vi "transfer char run_subvi_14_2014 05 30_JWa.vi"(0 "VISA session":refnum<visa-resource-name>="GPIB0::17::INSTR", 1 "Y2 axis settings":T7={"Y2 axis on/off"=FALSE, "MINIMUM"=0.0, "MAXIMUM"=1.0, "Variable name"="Ig", "LIN or LOG axis"="LIN"} {"MAXIMUM" format="%.9f"; "MINIMUM" format="%.9f"}, 3 "LKG Path":path, 5 "Var1 sweep settings":T9={"start"=40.0, "stop"=-40.0, "step (linear only)"=-1.0, "sweep spacing (linear: 0)"=0, "sweep mode"=FALSE, "compliance (V)"=100.0, "compliance (A)"=0.001} {"compliance (A)" format="%^.2e"; "compliance (V)" format="%.2f"; "sweep spacing (linear: 0)" items=["linear", "log 10", "log 25", "log 50"]; "step (linear only)" format="%.2f"; "stop" format="%.2f"; "start" format="%.2f"}, 7 "Var2 step settings":T8={"compliance (A)"=0.001, "compliance (V)"=100.0, "start"=-2.0, "total points"=2, "step"=-38.0} {"step" format="%.2f"; "start" format="%.2f"; "compliance (V)" format="%.2f"; "compliance (A)" format="%^.2e"}, 9 "integration time":u32(slide) scale=0.0..2.0, 10 "SMU Config":T2={"Vname"="Vs", "Vname 2"="Vd", "Vname 3"="Vg", "Vname 4"="V4", "Iname"="Is", "Iname 2"="Id", "Iname 3"="Ig", "Iname 4"="I4", "Mode"=4, "Mode 2"=0, "Mode 3"=0, "Mode 4"=0, "Function"=4, "Function 2"=2, "Function 3"=1, "Function 4"=4, "Value (V or A)"=0.0, "Value (Either V or A) 2"=0.0, "Value (Either V or A) 3"=0.0, "Value (Either V or A) 4"=0.0} {"Function" items=["disabled", "Var1", "Var2", "Var1'", "Constant"]; "Mode" items=["V", "I", "VPulse", "IPulse", "Common"]; "Function 4" items=["disabled", "Var1", "Var2", "Var1'", "Constant"]; "Mode 4" items=["V", "I", "VPulse", "IPulse", "Common"]; "Function 3" items=["disabled", "Var1", "Var2", "Var1'", "Constant"]; "Mode 3" items=["V", "I", "VPulse", "IPulse", "Common"]; "Function 2" items=["disabled", "Var1", "Var2", "Var1'", "Constant"]; "Mode 2" items=["V", "I", "VPulse", "IPulse", "Common"]}, 11 "Input Path":path, 12 "Dielectric Constant":dbl=5.0, 13 "Sample Properties:":T6 {"Date Created" format="%<%x>T"}, 14 "Ambient Temp (Y/N)":bool=TRUE, 15 "Error In":errorcluster) -> (2 "Check Cluster":T4, 4 "Output":T5 {"Mobility-Lin" format="%#_4e"; "Mobility-Sat" format="%#_4e"}, 6 "Graph Cluster":T3, 8 "Error Out":errorcluster)   [LabVIEW 2012]
panel:
  in  "Y1 Axis Settings":T1={"Y1 axis"="Id", "MINIMUM"=-1e-05, "MAXIMUM"=0.0, "LIN or LOG axis"="LIN"} {"MAXIMUM" format="%.2e"; "MINIMUM" format="%_2e"}
  out "Output Path":path
  in  "NumPts":dbl=5.0
  out "Gate Current Plot":cluster{"trace":dbl[], "trace":dbl[]}(graph)
  out "graphic display":cluster{"trace":dbl[], "trace":dbl[]}(graph)
  in  "wait time parameter":dbl=1.0
  in  "compliance (A)":dbl=0.001 format="%^.2e"
  in  "compliance (V)":dbl=100.0 format="%^.2e"
  in  "reset":bool=TRUE
  # "SMU1"
  # "SMU2"
  # "SMU3"
  # "SMU4"
  # "Sample Properties:"
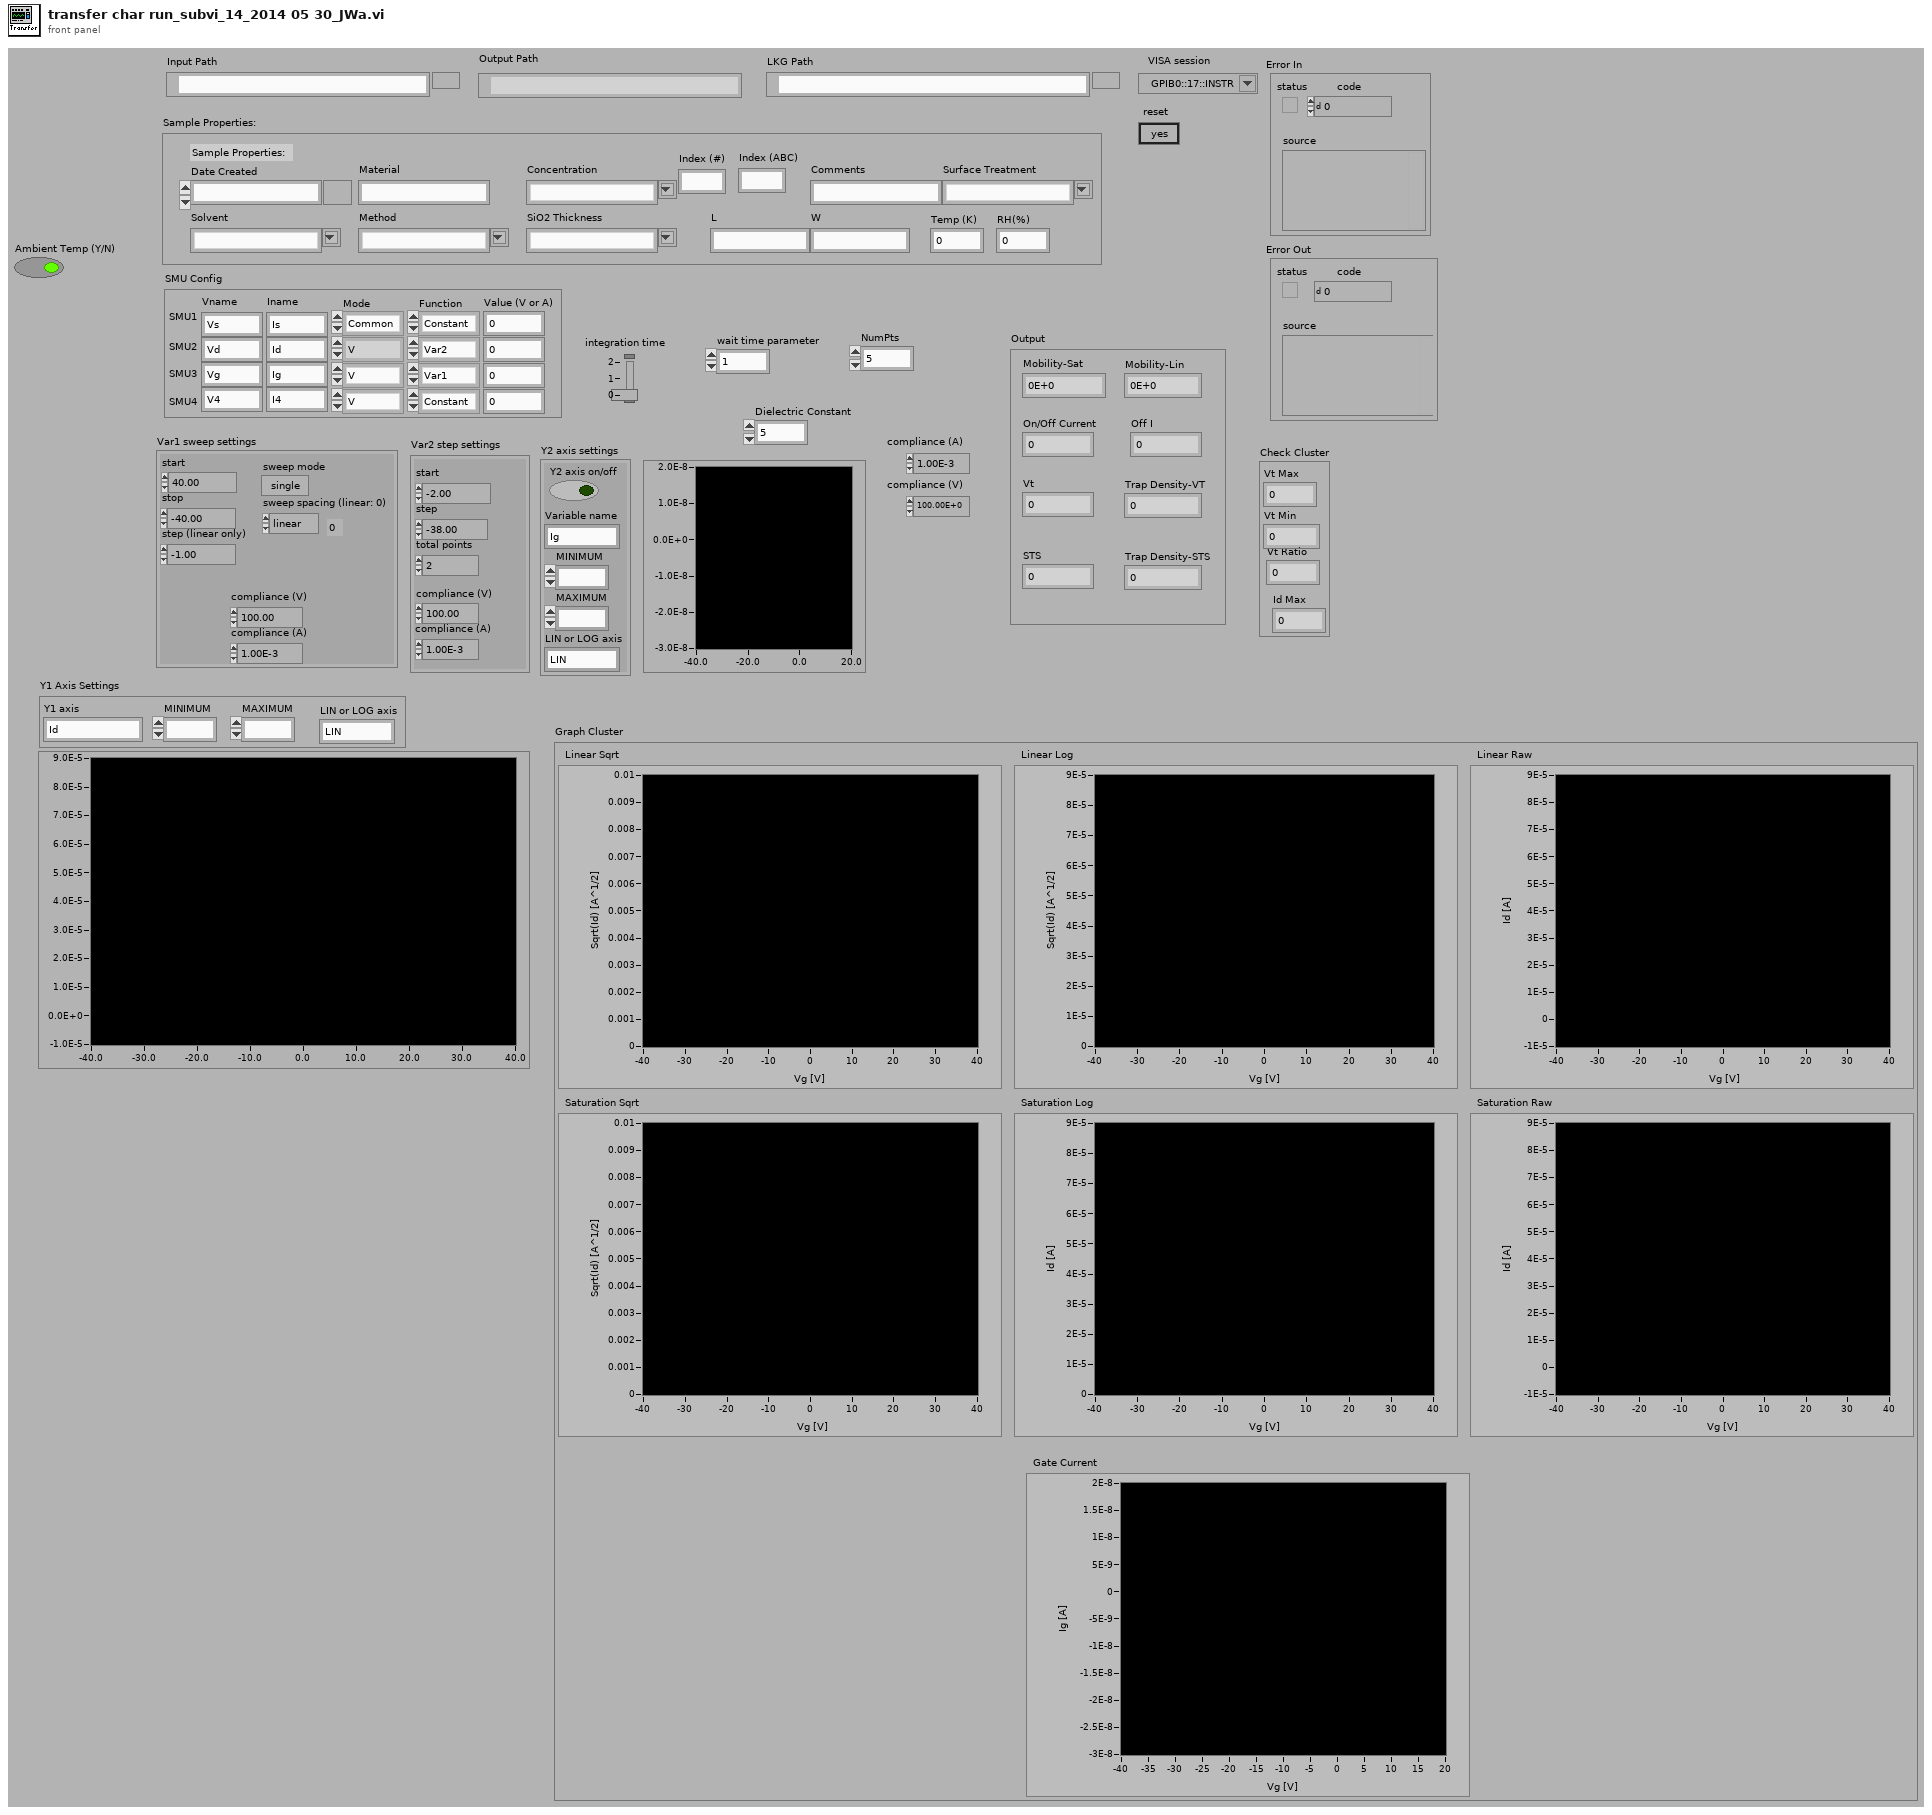
[diagram p1: front panel]
types:
  T1 = cluster{"Y1 axis":string, "MINIMUM":ext, "MAXIMUM":ext, "LIN or LOG axis":string}
  T2 = cluster{"Vname":string, "Vname 2":string, "Vname 3":string, "Vname 4":string, "Iname":string, "Iname 2":string, "Iname 3":string, "Iname 4":string, "Mode":u16, "Mode 2":u16, "Mode 3":u16, "Mode 4":u16, "Function":u16, "Function 2":u16, "Function 3":u16, "Function 4":u16, "Value (V or A)":dbl, "Value (Either V or A) 2":dbl, "Value (Either V or A) 3":dbl, "Value (Either V or A) 4":dbl}
  T3 = cluster{"Linear Sqrt":cluster{dbl[], "trace":dbl[]}[], "Linear Log":cluster{dbl[], "trace":dbl[]}[], "Linear Raw":cluster{dbl[], dbl[]}[], "Saturation Sqrt":cluster{dbl[], "trace":dbl[]}[], "Saturation Log":cluster{dbl[], "trace":dbl[]}[], "Saturation Raw":cluster{dbl[], "trace":dbl[]}[], "Gate Current":cluster{dbl[], "trace":dbl[]}[]}
  T4 = cluster{"Vt Max":i32, "Vt Min":i32, "Vt Ratio":i32, "Id Max":dbl}
  T5 = cluster{"Mobility-Sat":dbl, "Mobility-Lin":dbl, "On/Off Current":dbl, "Off I":dbl, "Vt":dbl, "STS":dbl, "Trap Density-VT":dbl, "Trap Density-STS":dbl}
  T6 = cluster{"Date Created":timestamp, "Material":string, "Solvent":string, "Concentration":string, "Method":string, "SiO2 Thickness":string, "Index (#)":string, "Index (ABC)":string, "L":string, "W":string, "Surface Treatment":string, "Comments":string, "Temp (K)":dbl, "RH(%)":dbl}
  T7 = cluster{"Y2 axis on/off":bool, "MINIMUM":ext, "MAXIMUM":ext, "Variable name":string, "LIN or LOG axis":string}
  T8 = cluster{"compliance (A)":dbl, "compliance (V)":dbl, "start":dbl, "total points":u16, "step":dbl}
  T9 = cluster{"start":dbl, "stop":dbl, "step (linear only)":dbl, "sweep spacing (linear: 0)":u16, "sweep mode":bool, "compliance (V)":dbl, "compliance (A)":dbl}
  T10 = cluster{"spreadsheet string":string, "spreadsheet string":string, "spreadsheet string":string}
  T11 = cluster{"Mobility-Sat":dbl, "Mobility-Lin":dbl, "On/Off I-Sat":dbl, "Off I-Sat":dbl, "VT-Sat":dbl, "Sub Threshold Swing":dbl, "Trap Density-VT":dbl, "Trap Density (N)":dbl}
  T12 = cluster{"Vt Max":dbl, "Vt Min":dbl, "Vt Ratio":dbl, "Id Max":dbl}
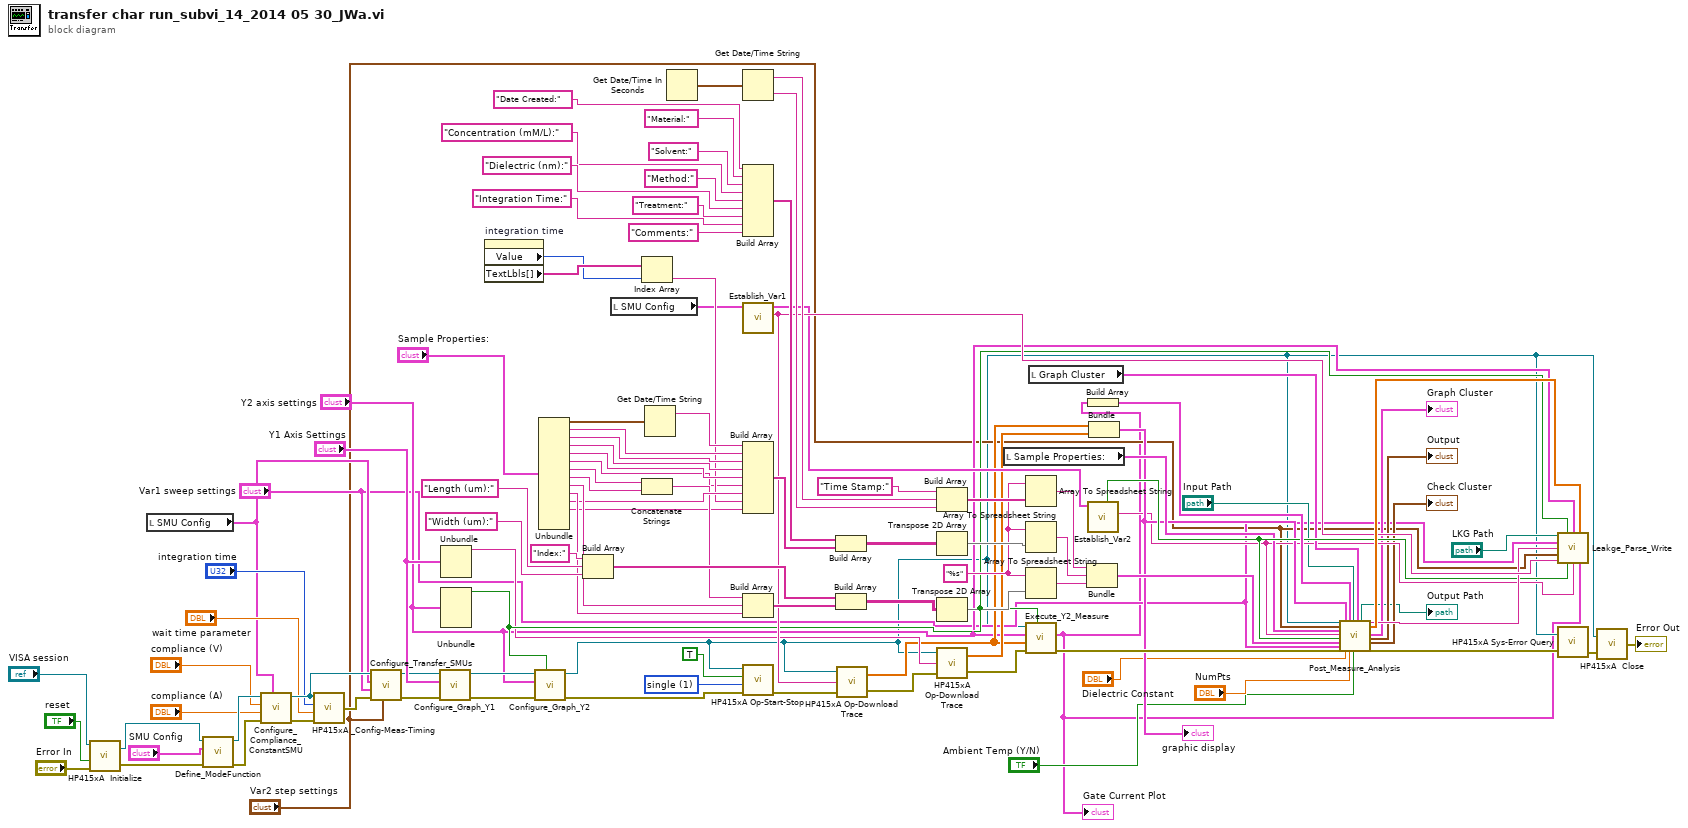
[diagram p0: block diagram]
diagram:
  w47 = u32 1 items=["stop  ", "single  ", "single-append  ", "stress start  ", "continuous  ", "standby on  ", "standby off  ", "zero  "] ("function (stop:0)")
  w69 = "%s"
  n1 = call "HP415xA  Initialize.vi"("instrument descriptor"="VISA session", "reset"="reset", "error in (no error)"="Error In") -> ("VISA session"=w55:refnum<visa-resource-name>, "error out"=w57:errorcluster)  [unwired: 2 in]
  n2 = local read "SMU Config"() -> (w6:T2)
  n3 = call "Define_ModeFunction.vi"("error in (no error)"=w57, "SMU Config"="SMU Config", "VISA Refnum in"=w55) -> ("error out"=w58:errorcluster, "VISA Refnum out"=w60:refnum<visa-resource-name>)  [unwired: 7 in]
  n4 = call "Configure_Compliance_ConstantSMU.vi"("SMU Config"=w6, "error in (no error)"=w58, "compliance (A)"="compliance (A)", "compliance (V)"="compliance (V)", "VISA In"=w60) -> ("error out"=w59:errorcluster, "VISA Out"=w61:refnum<visa-resource-name>)  [unwired: 5 in]
  n5 = call "HP415xA _Config-Meas-Timing.vi"("error in (no error)"=w59, "wait time parameter"="wait time parameter", "integration time"="integration time", "VISA session"=w61) -> ("error out"=w56:errorcluster)  [unwired: 2 in]
  n6 = call "Configure_Transfer_SMUs.vi"("Var2 step settings"="Var2 step settings", "error in (no error)"=w56, "Var1 sweep settings"="Var1 sweep settings", "SMU Config"=w6, "VISA In"=w61) -> ("error out"=w21:errorcluster, "VISA Out"=w3:refnum<visa-resource-name>)  [unwired: 5 in]
  n7 = call "Configure_Graph_Y1.vi"("error in (no error)"=w21, "Y1 Axis Settings"="Y1 Axis Settings", "VISA In"=w3) -> ("error out"=w44:errorcluster, "VISA Out"=w31:refnum<visa-resource-name>)  [unwired: 7 in]
  n8 = Unbundle("Y1 Axis Settings") -> ("Y1 axis"=w33:string)  [unwired: 3 out]
  n9 = Unbundle("Y2 axis settings") -> ("Y2 axis on/off"=w34:bool)  [unwired: 4 out]
  n10 = property on="integration time" class="Slide (strict)"() -> ("Value"=w64:u32, "TextLbls[]"=w65:string[])  [unwired: 2 in, 2 out]
  n11 = call "Configure_Graph_Y2.vi"("Execute?"=w34, "error in (no error)"=w44, "Y2 axis settings"="Y2 axis settings", "VISA In"=w31) -> ("error out"=w45:errorcluster, "VISA Out"=w2:refnum<visa-resource-name>)  [unwired: 6 in]
  n12 = Unbundle("Sample Properties:") -> ("Date Created"=w81:timestamp, "Material"=w80:string, "Solvent"=w77:string, "Concentration"=w76:string, "Method"=w79:string, "SiO2 Thickness"=w51:string, "Index (#)"=w72:string, "Index (ABC)"=w71:string, "L"=w74:string, "W"=w75:string, "Surface Treatment"=w73:string, "Comments"=w66:string)  [unwired: 2 out]
  n13 = Build Array("Index:", "Length (um):", "Width (um):") -> (w87:string[])
  n14 = local read "SMU Config"() -> (w62:T2)
  n15 = Index Array(array=w65, index=w64) -> (element=w63:string)
  n16 = Concatenate Strings(w72, w71) -> (w70:string)
  n17 = Get Date/Time String(seconds (now)=w81) -> (date string=w107:string)  [unwired: 2 in, 1 out]
  n18 = Get Date/Time In Seconds() -> (seconds since 1Jan1904=w102:timestamp)
  n19 = Get Date/Time String(seconds (now)=w102) -> (date string=w101:string, time string=w100:string)  [unwired: 2 in]
  n20 = Build Array("Date Created:", "Material:", "Solvent:", "Concentration (mM/L):", "Method:", "Dielectric (nm):", "Treatment:", "Integration Time:", "Comments:") -> (w91:string[])
  n21 = call "Establish_Var1.vi"("SMU Config In"=w62) -> ("Vname"=w38:string, "SMU Config Out"=w35:T2)  [unwired: 8 in]
  n22 = Build Array(w107, w80, w77, w76, w79, w51, w73, w63, w66) -> (w90:string[])
  n23 = Build Array(w70, w74, w75) -> (w86:string[])
  n24 = call "HP415xA Op-Start-Stop.vi"("error in (no error)"=w45, "function (stop:0)"=w47, "wait until finish"=TRUE, "VISA session"=w2) -> ("error out"=w46:errorcluster)  [unwired: 6 in, 1 out]
  n25 = Build Array(w91, w90) -> (w89:string[][])
  n26 = Build Array(w87, w86) -> (w85:string[][])
  n27 = call "HP415xA Op-Download Trace.vi"("error in (no error)"=w46, "trace (variable) name"=w38, "VISA session"=w2) -> ("error out"=w50:errorcluster, "trace"=w26:dbl[])
  n28 = Build Array("Time Stamp:", w101, w100) -> (w99:string[])
  n29 = Transpose 2D Array(2D array=w89) -> (transposed array=w88:string[][])
  n30 = Transpose 2D Array(2D array=w85) -> (transposed array=w84:string[][])
  n31 = call "HP415xA Op-Download Trace.vi"("error in (no error)"=w50, "trace (variable) name"=w33, "VISA session"=w2) -> ("error out"=w43:errorcluster, "trace"=w28:dbl[])
  n32 = local read "Sample Properties:"() -> (w29:T6)
  n33 = Array To Spreadsheet String(array=w99, 3:w69) -> (spreadsheet string=w92:string)  [unwired: 1 in]
  n34 = Array To Spreadsheet String(array=w88, 3:w69) -> (spreadsheet string=w95:string)  [unwired: 1 in]
  n35 = Array To Spreadsheet String(array=w84, 3:w69) -> (spreadsheet string=w83:string)  [unwired: 1 in]
  n36 = call "Execute_Y2_Measure.vi"("VISA In"=w2, "Y2 axis settings"="Y2 axis settings", "X-Axis Trace"=w26, "error in (no error)"=w43, "Y2 axis on/off"=w34) -> ("Y2 Output Cluster"=w1:cluster{"trace":dbl[], "trace":dbl[]}, "error out"=w40:errorcluster)  [unwired: 4 in]
  "Gate Current Plot" <- w1
  n37 = local read "Graph Cluster"() -> (w24:T3)
  n38 = Bundle("spreadsheet string"=w92, "spreadsheet string"=w95, "spreadsheet string"=w83) -> (w30:T10)  [unwired: 1 in]
  n39 = Build Array(w1) -> (w39:cluster{"trace":dbl[], "trace":dbl[]}[])
  n40 = call "Establish_Var2.vi"("SMU Config In"=w35) -> ("Vname"=w23:string, "Execute?"=w36:bool)  [unwired: 8 in, 1 out]
  n41 = Bundle("trace"=w26, "trace"=w28) -> (w27:cluster{"trace":dbl[], "trace":dbl[]})  [unwired: 1 in]
  "graphic display" <- w27
  n42 = call "Post_Measure_Analysis.vi"("VISA Refnum in"=w2, "Var2 step settings"="Var2 step settings", "Sample Properties:"=w29, "Vname"=w23, "Execute?"=w36, "Header Strings"=w30, "Var1 sweep settings"="Var1 sweep settings", "error in (no error)"=w40, "Id Vg Data"=w27, "Dielectric Constant"="Dielectric Constant", "Gate Current"=w39, "NumPts"="NumPts", "Input Path"="Input Path", "Ambient Temp (Y/N)"="Ambient Temp (Y/N)", "Graph Cluster in"=w24) -> ("File out"=→"Output Path":path, "Header out"=w37:string, "Vd Data"=w41:dbl[], "Graph Cluster out"=→"Graph Cluster":T3, "Device Properties Out"=→"Output":T11, "Check Cluster"=→"Check Cluster":T12, "error out"=w42:errorcluster)  [unwired: 4 in, 2 out]
  n43 = call "Leakge_Parse_Write.vi"("LKG Path"="LKG Path", "Y2 axis on/off"=w34, "Y2 axis settings"="Y2 axis settings", "Vd Data"=w41, "Var1 sweep settings"="Var1 sweep settings", "Header in"=w37, "Var2 step settings"="Var2 step settings", "Vname 2"=w38, "Execute?"=w36, "Vname"=w23, "Y2 Output Cluster"=w1) -> ()  [unwired: 5 in]
  n44 = call "HP415xA Sys-Error Query.vi"("VISA session"=w2, "error in (no error)"=w42) -> ("error out"=w49:errorcluster)  [unwired: 2 in, 1 out]
  n45 = call "HP415xA  Close.vi"("error in (no error)"=w49, "VISA session"=w2) -> ("error out"=→"Error Out":errorcluster)
